vi "PID Control.vi"() -> ()   [LabVIEW 2024]
uses:
  <vilib>/addons/control/pid/pid.llb/PID Advanced (DBL).vi
  <vilib>/addons/control/pid/NI_PID_pid.lvlib
panel:
  in  "Type of Controller":u16(ring)=2 items=["P", "PI", "PID"]
  out "PID Output":dbl format="%.2f"
  in  "Setpoint Value":dbl format="%#_13g"
  in  "Motor Sensor":dbl format="%#_13g"
  # "iHPU PID Control"
  # "* This will be read back"
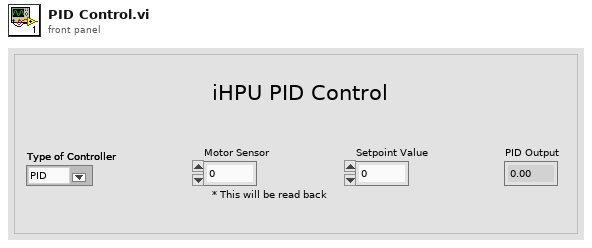
[diagram p1: front panel]
types:
  T1 = cluster{"proportional gain (Kc)":dbl, "integral time (Ti, min)":dbl, "derivative time (Td, min)":dbl}
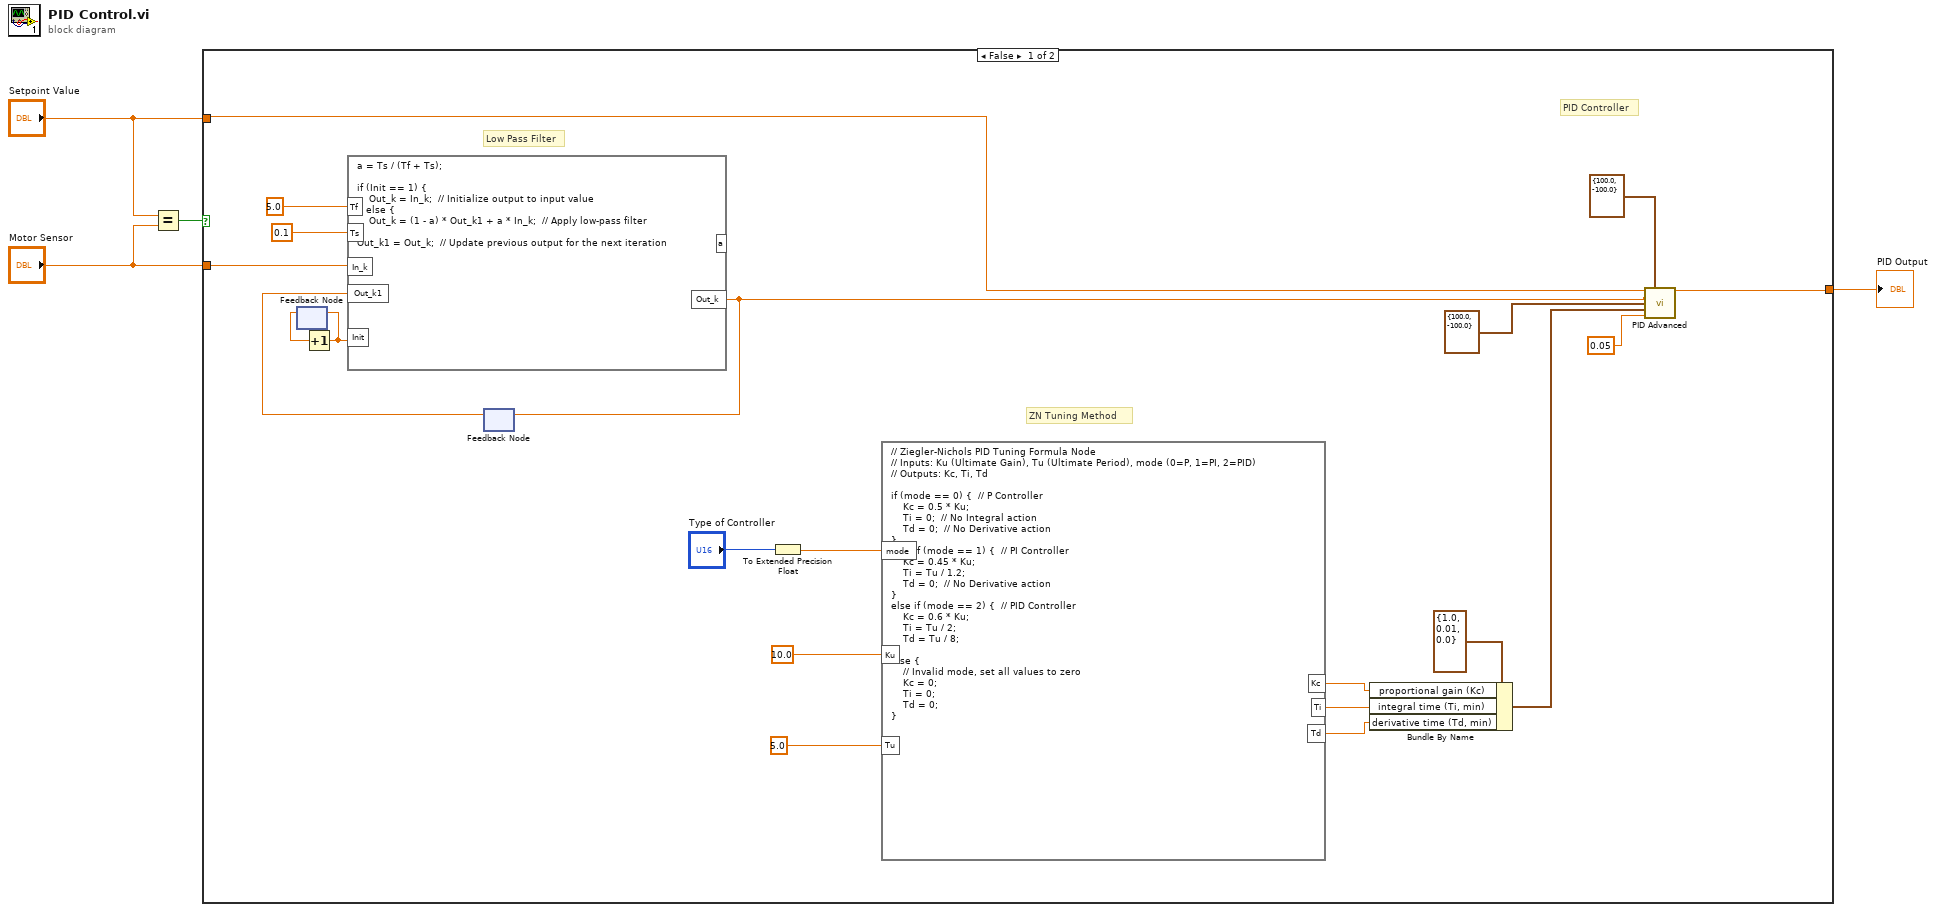
[diagram p0: block diagram]
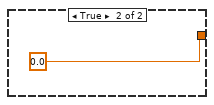
[diagram p2: hidden frame]
diagram:
  n1 = Equal?(x="Setpoint Value", y="Motor Sensor") -> (x = y?=w4:bool)
  n2 = case shown="False" w4 {
    tunnel: "Motor Sensor" -> [w11 _]
    tunnel: "Setpoint Value" -> [w10 _]
    tunnel: [w9 0.0 ("output")] -> w1
    frame False {
      # "PID Controller"
      # "ZN Tuning Method"
      # "Low Pass Filter"
      n3 = feedback #1() -> (w12:dbl)  [unwired: 1 in]
      n4 = Increment(x=w12) -> (x+1=w13:dbl)
      n5 = feedback-in #1(w13) -> ()
      n6 = feedback #2() -> (w15:dbl)  [unwired: 1 in]
      n7 = formula code="a = Ts / (Tf + Ts);\n\nif (Init == 1) {\n    Out_k = In_k;  // Initialize output to input value\n} else {\n    Out_k = (1 - a) * Out_k1 + a * In_k;  // Apply low-pass filter\n}\nOut_k1 = Out_k;  // Update previous output for the next iteration"("Out_k1"=w15, "In_k"=w11, "Ts"=0.1, "Tf"=5.0, "Init"=w13) -> ("Out_k"=w14:dbl)  [unwired: 1 out]
      n8 = feedback-in #2(w14) -> ()
      n9 = To Extended Precision Float(1:"Type of Controller") -> (0:w6:ext)
      n10 = formula code="// Ziegler-Nichols PID Tuning Formula Node\n// Inputs: Ku (Ultimate Gain), Tu (Ultimate Period), mode (0=P, 1=PI, 2=PID)\n// Outputs: Kc, Ti, Td\n\nif (mode == 0) {  // P Controller\n    Kc = 0.5 * Ku;\n    Ti = 0;  // No Integral action\n    Td = 0;  // No Derivative action\n}\nelse if (mode == 1) {  // PI Controller\n    Kc = 0.45 * Ku;\n    Ti = Tu / 1.2;\n    Td = 0;  // No Derivative action\n}\nelse if (mode == 2) {  // PID Controller\n    Kc = 0.6 * Ku;\n    Ti = Tu / 2;\n    Td = Tu / 8;\n}\nelse {\n    // Invalid mode, set all values to zero\n    Kc = 0;\n    Ti = 0;\n    Td = 0;\n}"("mode"=w6, "Ku"=10.0 ("input variable 2"), "Tu"=5.0 ("input variable 3")) -> ("Kc"=w19:dbl, "Ti"=w18:dbl, "Td"=w17:dbl)
      n11 = Bundle By Name(cluster=T1 {"proportional gain (Kc)"=1.0, "integral time (Ti, min)"=0.01, "derivative time (Td, min)"=0.0} ("PID gains"), "proportional gain (Kc)"=w19, "integral time (Ti, min)"=w18, "derivative time (Td, min)"=w17) -> (w16:T1)
      n12 = call-poly <vilib>:"PID Advanced.vi"("setpoint"=w10, "output range"=cluster{"Output high":dbl, "Output low":dbl} {"Output high"=100.0, "Output low"=-100.0} ("Controller output (u)\nrange [V] 3"), "process variable"=w14, "setpoint range"=cluster{"Setpoint high":dbl, "Setpoint low":dbl} {"Setpoint high"=100.0, "Setpoint low"=-100.0} ("Setpoint (y_SP)\nrange [kRPM] 3"), "PID gains"=w16, "dt (s)"=0.05 ("Time step Ts [s] 3")) -> ("output"=w9:dbl)  [unwired: 8 in, 1 out]
    }
    frame True {
    }
  }
  "PID Output" <- w1
